vi "Get Cache File Details.vi"(8 "error in (no error)":errorcluster, 11 "WorkSpace / Repo path":path) -> (0 "error out":errorcluster, 1 "Cache Found?":bool, 2 "Create cache?":bool, 3 "Cache file name":path)   [LabVIEW 2019, in "Hawkeye.lvlib"]
uses:
  Hawkeye.lvlib
  <userlib>/_OpenG.lib/file/file.llb/Valid Path - Traditional__ogtk.vi
  <userlib>/_OpenG.lib/file/file.llb/File Exists - Scalar__ogtk.vi
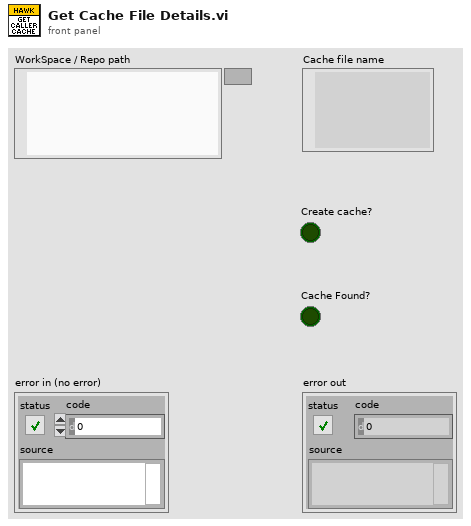
[diagram p1: front panel]
types:
  T1 = enum16{"open", "replace", "create", "open or create", "replace or create", "replace or create with confirmation"}
  T2 = typedef "Hawkeye.lvlib/HawkeyePathConfigs.ctl" = cluster{"GlobalIncludePaths":path[], "GlobalExcludePaths":path[], "BuildSpecsIncludePaths":path[], "ActualDepsIncludePaths":path[], "WorkspacePath":path, "SourceFolderPaths":path[], "ChangedFilesLogpaths":map{string, path}, "CacheRecreateDuration":dbl}
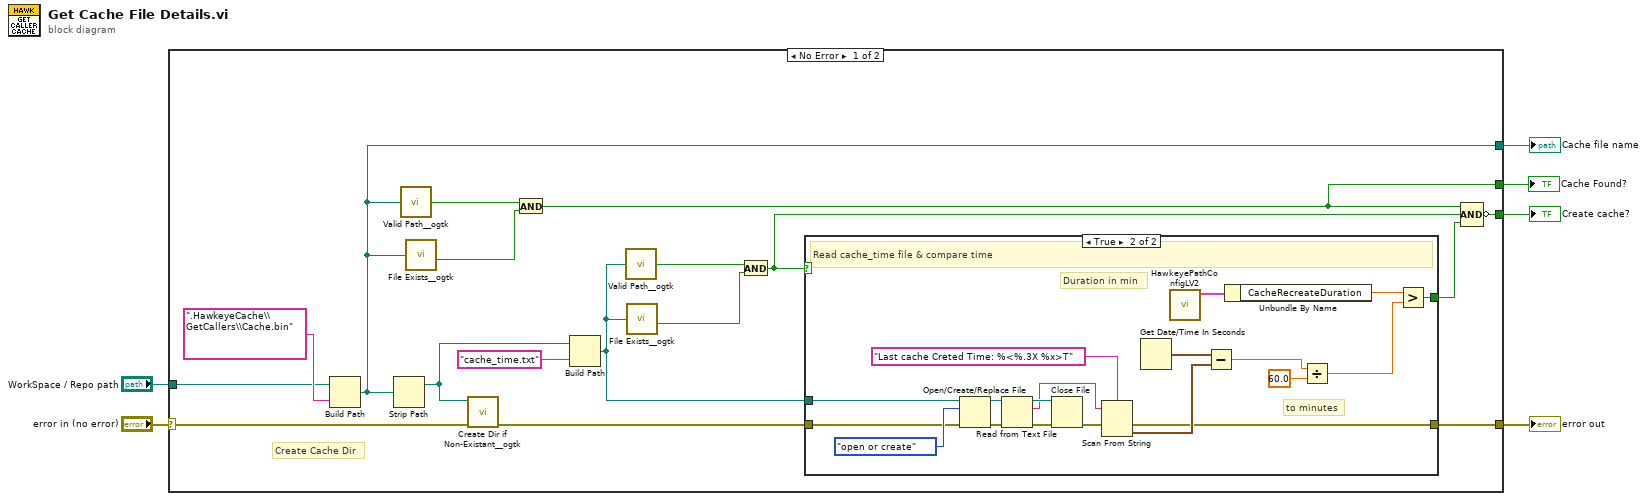
[diagram p0: block diagram]
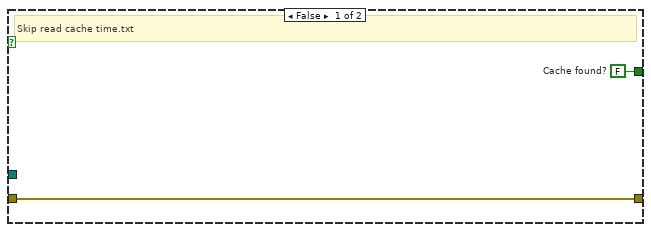
[diagram p2: hidden frame]
diagram:
  n1 = case shown="No Error" "error in (no error)" {
    selector: "error in (no error)" -> [w22 w45]
    tunnel: "WorkSpace / Repo path" -> [w21 _]
    tunnel: [w20 _] -> w4
    tunnel: [w10 _] -> w3
    tunnel: [w9 w45] -> w2
    tunnel: [w7 _] -> w1
    frame No Error {
      # "Create Cache Dir"
      n2 = Build Path(base path=w21, name or relative path=".HawkeyeCache\\GetCallers\\Cache.bin") -> (appended path=w20:path)
      n3 = Strip Path(path=w20) -> (stripped path=w19:path)  [unwired: 1 out]
      n4 = call-poly <userlib>:"Valid Path__ogtk.vi"("path"=w20) -> ("valid"=w15:bool)
      n5 = call-poly <userlib>:"File Exists__ogtk.vi"("file path"=w20) -> ("exists"=w14:bool)  [unwired: 6 in, 1 out]
      n6 = call <userlib>:"Create Dir if Non-Existant__ogtk.vi"("error in (no error)"=w22, "Directory Path"=w19) -> ("error out"=w12:errorcluster)  [unwired: 7 in, 2 out]
      n7 = And(x=w15, y=w14) -> (x .and. y?=w7:bool)
      n8 = Build Path(base path=w19, name or relative path="cache_time.txt") -> (appended path=w13:path)
      n9 = call-poly <userlib>:"Valid Path__ogtk.vi"("path"=w13) -> ("valid"=w17:bool)
      n10 = call-poly <userlib>:"File Exists__ogtk.vi"("file path"=w13) -> ("exists"=w16:bool)  [unwired: 6 in, 1 out]
      n11 = And(x=w17, y=w16) -> (x .and. y?=w8:bool)
      n12 = case shown="True" w8 {
        tunnel: w13 -> [_ w39]
        tunnel: w12 -> [w24 w38]
        tunnel: [w25 w33] -> w11
        tunnel: [w24 w31] -> w9
        frame False {
          w25 = FALSE  # Cache found?
          # "Skip read cache time.txt"
        }
        frame True {
          # "Duration in min"
          # "to minutes"
          # "Read cache_time file & compare time"
          n13 = Open/Create/Replace File(file path (use dialog)=w39, error in=w38, operation (0:open)=T1."open or create") -> (refnum out=w44:refnum<file>, error out=w41:errorcluster)  [unwired: 3 in, 1 out]
          n14 = Read from Text File(file (use dialog)=w44, error in=w41) -> (refnum out=w43:refnum<file>, text=w37:string, error out=w42:errorcluster)  [unwired: 2 in, 1 out]
          n15 = Close File(refnum=w43, error in=w42) -> (error out=w30:errorcluster)  [unwired: 1 out]
          n16 = Scan From String(format string="Last cache Creted Time: %<%.3X %x>T" ("name or relative path"), input string=w37, error in=w30) -> (error out=w31:errorcluster, output 1=w35:timestamp)  [unwired: 2 in, 2 out]
          n17 = Get Date/Time In Seconds() -> (seconds since 1Jan1904=w32:timestamp)
          n18 = call "HawkeyePathConfigLV2.vi"() -> ("Hawkeye Path Config Out"=w36:T2)  [unwired: 11 in]
          n19 = Subtract(x=w32, y=w35) -> (x-y=w27:dbl)
          n20 = Unbundle By Name(w36) -> ("CacheRecreateDuration"=w34:dbl)
          n21 = Divide(x=w27, y=60.0) -> (x/y=w26:dbl)
          n22 = Greater?(x=w34, y=w26) -> (0:w33:bool)
        }
      }
      n23 = Compound Arithmetic op=AND(w7, w8, w11) -> (invert w10:bool)
    }
    frame Error {
    }
  }
  "error out" <- w2
  "Cache file name" <- w4
  "Create cache?" <- w3
  "Cache Found?" <- w1
